vi "Get Match Score.vi"(8 "Error In":errorcluster, 10 "Number of Matches":i32, 11 "Matches (real-world)":T1[](array[typedef]) {"Correlation Score" format="%.2f"; "Target Template Curve Score" format="%.2f"; "Template Target Curve Score" format="%.2f"; "Bounding Box"."y" format="%.2f"; "Bounding Box"."x" format="%.2f"; "Position"."y" format="%.2f"; "Position"."x" format="%.2f"; "Score" format="%.2f"; "Scale" format="%.2f"; "Angle" format="%.2f"; "Occlusion %" format="%.2f"}) -> (0 "Error Out":errorcluster, 2 "Position":cluster{"x":sgl, "y":sgl}, 3 "Score":sgl)   [LabVIEW 2018]
uses:
  <vilib>/vision/Pattern Matching.llb/IMAQ GM Match Report.ctl
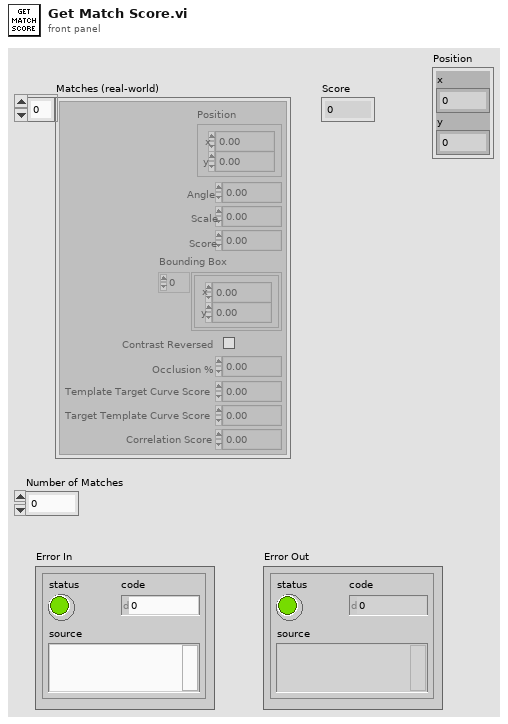
[diagram p1: front panel]
types:
  T1 = typedef "IMAQ GM Match Report.ctl" = cluster{"Position":cluster{"x":sgl, "y":sgl}, "Angle":sgl, "Scale":sgl, "Score":sgl, "Bounding Box":cluster{"x":sgl, "y":sgl}[], "Contrast Reversed":bool, "Occlusion %":sgl, "Template Target Curve Score":sgl, "Target Template Curve Score":sgl, "Correlation Score":sgl}
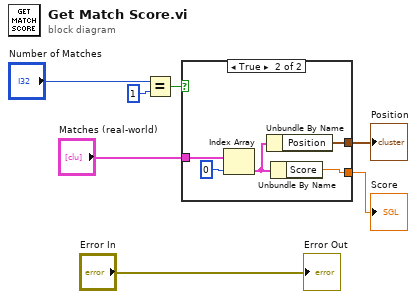
[diagram p0: block diagram]
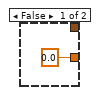
[diagram p2: hidden frame]
diagram:
  n1 = Equal?(x="Number of Matches", y=1) -> (x = y?=w5:bool)
  n2 = case shown="True" w5 {
    tunnel: "Matches (real-world)" -> [_ w13]
    tunnel: [sgl 0.0 ("Score") w11] -> w7
    tunnel: [_ w9] -> w2
    frame False {
    }
    frame True {
      n3 = Index Array(array=w13, index=0) -> (element=w10:T1)
      n4 = Unbundle By Name(w10) -> ("Position"=w9:cluster{"x":sgl, "y":sgl})
      n5 = Unbundle By Name(w10) -> ("Score"=w11:sgl)
    }
  }
  "Score" <- w7
  "Position" <- w2
  "Error Out" <- "Error In"
